vi "Close Worksheet.vi"(8 "error in (no error)":errorcluster, 11 "worksheet in":refnum<class "worksheet.lvclass">) -> (0 "error out":errorcluster)   [LabVIEW 2017, in "Excel_Specific.lvlib" / "worksheet.lvclass"]
uses:
  worksheet.lvclass
  worksheet.lvclass/worksheet.ctl
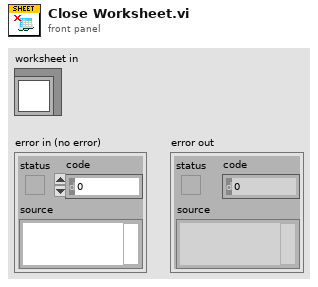
[diagram p1: front panel]
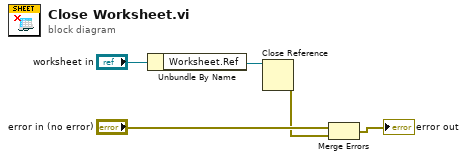
[diagram p0: block diagram]
diagram:
  n1 = Unbundle By Name("worksheet in") -> ("Worksheet.Ref"=w4:refnum<k24>)
  n2 = Close Reference(reference=w4) -> (error out=w1:errorcluster)  [unwired: 1 in]
  n3 = Merge Errors("error in (no error)", w1) -> (→"error out":errorcluster)
